vi "checkForTimeouts.vi"(8 "error in (no error)":errorcluster, 11 "ILCCommunications in":refnum<class "ILCCommunications.lvclass">) -> (0 "error out":errorcluster, 3 "ILCCommunications out":refnum<class "ILCCommunications.lvclass">)   [LabVIEW 2016, in "ILCCommunications.lvclass"]
uses:
  ILCCommunications.lvclass
  ILCCommunications.lvclass/ILCCommunications.ctl
  Common_RT_HPILC/HPILC/HPILC.lvclass/HPILC.ctl
  Common_RT_ILC/ILC/ILC.lvclass/ILC.ctl
  getHPs.vi
  Common_RT_ILC/ILC/getILCData.vi
  Common_RT_HPILC/HPILC/getHPData.vi
  Common_RT_HPILC/HPILC/HPILC.lvclass
  D:/Code/ts_M1M3Support/Common_RT_ILC/ILC/ILC.lvclass
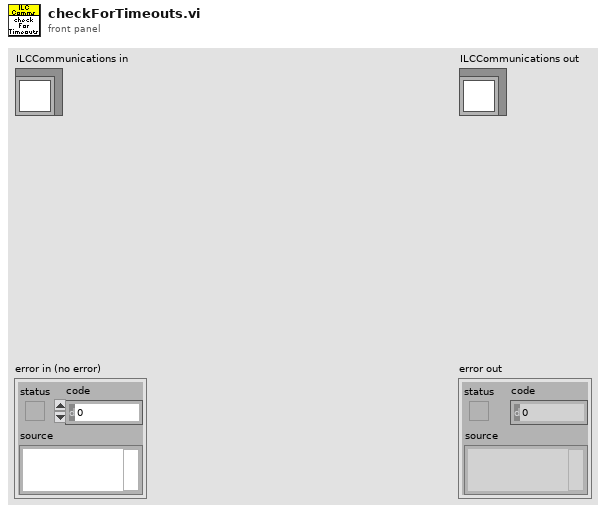
[diagram p1: front panel]
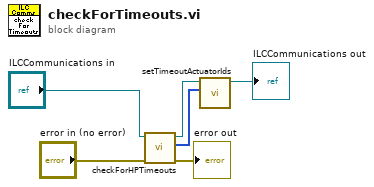
[diagram p0: block diagram]
diagram:
  n1 = call "checkForHPTimeouts.vi"("error in (no error)"="error in (no error)", "ILCCommunications in"="ILCCommunications in") -> ("error out"=→"error out":errorcluster, "IDs"=w1:i32[], "ILCCommunications out"=w3:refnum<class "ILCCommunications.lvclass">)  [unwired: 7 in]
  n2 = call "setTimeoutActuatorIds.vi"("TimeoutActuatorIds"=w1, "ILCCommunications in"=w3) -> ("ILCCommunications out"=→"ILCCommunications out":refnum<class "ILCCommunications.lvclass">)  [unwired: 9 in]
